vi "Table Select Section Paste.vi"(9 "Paste Value":string[][](array[string]), 11 "Table Ref In":refnum<vi>) -> (3 "Table Ref Out":refnum<vi>)   [LabVIEW 2024]
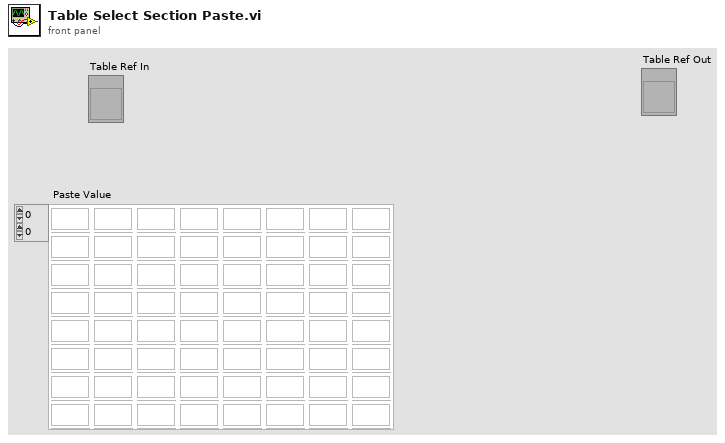
[diagram p1: front panel]
types:
  T1 = typedef "LVRowAndColumnTypeDef.ctl" = cluster{"Row":i32, "Column":i32}
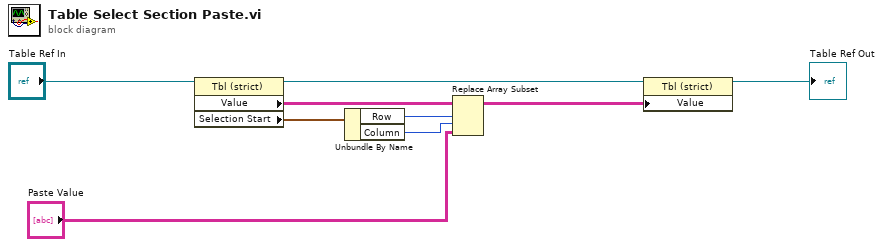
[diagram p0: block diagram]
diagram:
  n1 = property class="Tbl (strict)"(reference="Table Ref In") -> (reference out=w2:refnum<vi>, "Value"=w8:string[][], "Selection Start"=w9:T1)  [unwired: 1 in, 1 out]
  n2 = Unbundle By Name(w9) -> ("Row"=w7:i32, "Column"=w6:i32)
  n3 = Replace Array Subset(array=w8, new element="Paste Value", index (row)=w7, index (col)=w6) -> (w1:string[][])
  n4 = property class="Tbl (strict)"(reference=w2, "Value"=w1) -> (reference out=→"Table Ref Out":refnum<vi>)  [unwired: 1 in, 1 out]
